vi "Initialize Bank.vi"(9 "Bank Type":T1, 10 "Resources":T2, 11 "Bank in":refnum<class "Bank.lvclass">) -> (3 "Bank out":refnum<class "Bank.lvclass">)   [LabVIEW 2019, in "Bank.lvclass"]
uses:
  Bank.lvclass
  Bank Type.ctl
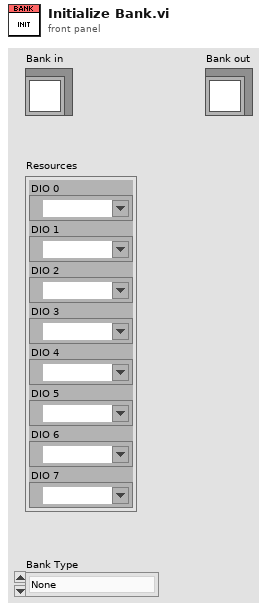
[diagram p1: front panel]
types:
  T1 = typedef "Bank Type.ctl" = enum16{"None", "Discrete Acquisition", "Discrete Generation", "PWM Acquisition", "PWM Generation"}
  T2 = cluster{"DIO 0":refnum<k21>, "DIO 1":refnum<k21>, "DIO 2":refnum<k21>, "DIO 3":refnum<k21>, "DIO 4":refnum<k21>, "DIO 5":refnum<k21>, "DIO 6":refnum<k21>, "DIO 7":refnum<k21>}
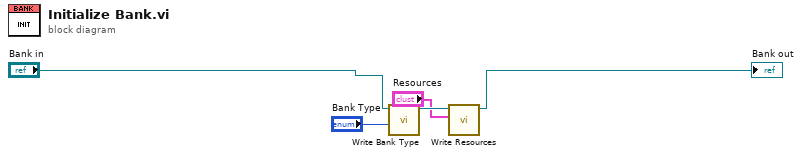
[diagram p0: block diagram]
diagram:
  n1 = call "Write Bank Type.vi"("Bank Type"="Bank Type", "Bank in"="Bank in") -> ("Bank out"=w4:refnum<class "Bank.lvclass">)  [unwired: 9 in]
  n2 = call "Write Resources.vi"("Resources"="Resources", "Bank in"=w4) -> ("Bank out"=→"Bank out":refnum<class "Bank.lvclass">)  [unwired: 9 in]
